vi "Generate Report work with Zee.vi"(6 "Graph Properties":T2(array[cluster])=[{"Plot Traces"=[{"Color Box"=4652800, "Boolean"=TRUE, "List 2"=5, "Boolean 2"=FALSE, "Boolean 3"=FALSE, "Offset"=0.0, "Gain"=1.0}, {"Color Box"=4467455, "Boolean"=TRUE, "List 2"=13, "Boolean 2"=TRUE, "Boolean 3"=FALSE, "Offset"=0.0, "Gain"=1.0}, {"Color Box"=16722474, "Boolean"=TRUE, "List 2"=21, "Boolean 2"=TRUE, "Boolean 3"=FALSE, "Offset"=0.0, "Gain"=1.0}], "Gain Calculations"={"Threshold Trace"=5, "Min Thresh/%"=0.2, "Max Thresh/%"=0.8, "Gain calculated by dividing"=13, "Gain Range"=enum."Best Est", "Pre-peak-ms"=30.0, "by"=5}, "Impulse Plane"=enum."Yaw", "Impulse Direction"=TRUE}, {"Plot Traces"=[{"Color Box"=4652800, "Boolean"=TRUE, "List 2"=5, "Boolean 2"=TRUE, "Boolean 3"=FALSE, "Offset"=0.0, "Gain"=1.0}, {"Color Box"=1966335, "Boolean"=TRUE, "List 2"=13, "Boolean 2"=FALSE, "Boolean 3"=FALSE, "Offset"=0.0, "Gain"=1.0}, {"Color Box"=16722474, "Boolean"=TRUE, "List 2"=21, "Boolean 2"=FALSE, "Boolean 3"=FALSE, "Offset"=0.0, "Gain"=1.0}], "Gain Calculations"={"Threshold Trace"=5, "Min Thresh/%"=0.2, "Max Thresh/%"=0.8, "Gain calculated by dividing"=13, "Gain Range"=enum."Best Est", "Pre-peak-ms"=30.0, "by"=5}, "Impulse Plane"=enum."Yaw", "Impulse Direction"=FALSE}, {"Plot Traces"=[{"Color Box"=4652800, "Boolean"=TRUE, "List 2"=5, "Boolean 2"=FALSE, "Boolean 3"=FALSE, "Offset"=0.0, "Gain"=1.0}, {"Color Box"=1966335, "Boolean"=TRUE, "List 2"=13, "Boolean 2"=TRUE, "Boolean 3"=FALSE, "Offset"=0.0, "Gain"=1.0}, {"Color Box"=16722474, "Boolean"=TRUE, "List 2"=21, "Boolean 2"=TRUE, "Boolean 3"=FALSE, "Offset"=0.0, "Gain"=1.0}], "Gain Calculations"={"Threshold Trace"=5, "Min Thresh/%"=0.2, "Max Thresh/%"=0.8, "Gain calculated by dividing"=21, "Gain Range"=enum."Best Est", "Pre-peak-ms"=30.0, "by"=5}, "Impulse Plane"=enum."Yaw", "Impulse Direction"=TRUE}, {"Plot Traces"=[{"Color Box"=4652800, "Boolean"=TRUE, "List 2"=5, "Boolean 2"=TRUE, "Boolean 3"=FALSE, "Offset"=0.0, "Gain"=1.0}, {"Color Box"=1966335, "Boolean"=TRUE, "List 2"=13, "Boolean 2"=FALSE, "Boolean 3"=FALSE, "Offset"=0.0, "Gain"=1.0}, {"Color Box"=16722474, "Boolean"=TRUE, "List 2"=21, "Boolean 2"=FALSE, "Boolean 3"=FALSE, "Offset"=0.0, "Gain"=1.0}], "Gain Calculations"={"Threshold Trace"=5, "Min Thresh/%"=0.2, "Max Thresh/%"=0.8, "Gain calculated by dividing"=21, "Gain Range"=enum."Best Est", "Pre-peak-ms"=30.0, "by"=5}, "Impulse Plane"=enum."Yaw", "Impulse Direction"=FALSE}, {"Plot Traces"=[{"Color Box"=4652800, "Boolean"=TRUE, "List 2"=4, "Boolean 2"=FALSE, "Boolean 3"=FALSE, "Offset"=0.0, "Gain"=1.0}, {"Color Box"=1966335, "Boolean"=TRUE, "List 2"=12, "Boolean 2"=TRUE, "Boolean 3"=FALSE, "Offset"=0.0, "Gain"=1.0}, {"Color Box"=16722474, "Boolean"=TRUE, "List 2"=20, "Boolean 2"=TRUE, "Boolean 3"=FALSE, "Offset"=0.0, "Gain"=1.0}], "Gain Calculations"={"Threshold Trace"=4, "Min Thresh/%"=0.2, "Max Thresh/%"=0.8, "Gain calculated by dividing"=12, "Gain Range"=enum."Best Est", "Pre-peak-ms"=30.0, "by"=4}, "Impulse Plane"=enum."Pitch", "Impulse Direction"=TRUE}, {"Plot Traces"=[{"Color Box"=4652800, "Boolean"=TRUE, "List 2"=4, "Boolean 2"=TRUE, "Boolean 3"=FALSE, "Offset"=0.0, "Gain"=1.0}, {"Color Box"=1966335, "Boolean"=TRUE, "List 2"=12, "Boolean 2"=FALSE, "Boolean 3"=FALSE, "Offset"=0.0, "Gain"=1.0}, {"Color Box"=16722474, "Boolean"=TRUE, "List 2"=20, "Boolean 2"=FALSE, "Boolean 3"=FALSE, "Offset"=0.0, "Gain"=1.0}], "Gain Calculations"={"Threshold Trace"=4, "Min Thresh/%"=0.2, "Max Thresh/%"=0.8, "Gain calculated by dividing"=12, "Gain Range"=enum."Best Est", "Pre-peak-ms"=30.0, "by"=4}, "Impulse Plane"=enum."Pitch", "Impulse Direction"=FALSE}, {"Plot Traces"=[{"Color Box"=4652800, "Boolean"=TRUE, "List 2"=4, "Boolean 2"=FALSE, "Boolean 3"=FALSE, "Offset"=0.0, "Gain"=1.0}, {"Color Box"=16860, "Boolean"=TRUE, "List 2"=12, "Boolean 2"=TRUE, "Boolean 3"=FALSE, "Offset"=0.0, "Gain"=1.0}, {"Color Box"=16716346, "Boolean"=TRUE, "List 2"=20, "Boolean 2"=TRUE, "Boolean 3"=FALSE, "Offset"=0.0, "Gain"=1.0}], "Gain Calculations"={"Threshold Trace"=4, "Min Thresh/%"=0.2, "Max Thresh/%"=0.8, "Gain calculated by dividing"=20, "Gain Range"=enum."Best Est", "Pre-peak-ms"=30.0, "by"=4}, "Impulse Plane"=enum."Pitch", "Impulse Direction"=TRUE}, {"Plot Traces"=[{"Color Box"=4652800, "Boolean"=TRUE, "List 2"=4, "Boolean 2"=TRUE, "Boolean 3"=FALSE, "Offset"=0.0, "Gain"=1.0}, {"Color Box"=4349695, "Boolean"=TRUE, "List 2"=12, "Boolean 2"=FALSE, "Boolean 3"=FALSE, "Offset"=0.0, "Gain"=1.0}, {"Color Box"=16716346, "Boolean"=TRUE, "List 2"=20, "Boolean 2"=FALSE, "Boolean 3"=FALSE, "Offset"=0.0, "Gain"=1.0}], "Gain Calculations"={"Threshold Trace"=4, "Min Thresh/%"=0.2, "Max Thresh/%"=0.8, "Gain calculated by dividing"=20, "Gain Range"=enum."Best Est", "Pre-peak-ms"=30.0, "by"=4}, "Impulse Plane"=enum."Pitch", "Impulse Direction"=FALSE}, {"Plot Traces"=[{"Color Box"=4652800, "Boolean"=TRUE, "List 2"=3, "Boolean 2"=FALSE, "Boolean 3"=FALSE, "Offset"=0.0, "Gain"=1.0}, {"Color Box"=4349695, "Boolean"=TRUE, "List 2"=11, "Boolean 2"=TRUE, "Boolean 3"=FALSE, "Offset"=0.0, "Gain"=1.0}, {"Color Box"=16716346, "Boolean"=TRUE, "List 2"=19, "Boolean 2"=TRUE, "Boolean 3"=FALSE, "Offset"=0.0, "Gain"=1.0}], "Gain Calculations"={"Threshold Trace"=3, "Min Thresh/%"=0.2, "Max Thresh/%"=0.8, "Gain calculated by dividing"=11, "Gain Range"=enum."Best Est", "Pre-peak-ms"=30.0, "by"=3}, "Impulse Plane"=enum."Roll", "Impulse Direction"=TRUE}, {"Plot Traces"=[{"Color Box"=4652800, "Boolean"=TRUE, "List 2"=3, "Boolean 2"=TRUE, "Boolean 3"=FALSE, "Offset"=0.0, "Gain"=1.0}, {"Color Box"=4349695, "Boolean"=TRUE, "List 2"=11, "Boolean 2"=FALSE, "Boolean 3"=FALSE, "Offset"=0.0, "Gain"=1.0}, {"Color Box"=16716346, "Boolean"=TRUE, "List 2"=19, "Boolean 2"=FALSE, "Boolean 3"=FALSE, "Offset"=0.0, "Gain"=1.0}], "Gain Calculations"={"Threshold Trace"=3, "Min Thresh/%"=0.2, "Max Thresh/%"=0.8, "Gain calculated by dividing"=11, "Gain Range"=enum."Best Est", "Pre-peak-ms"=30.0, "by"=3}, "Impulse Plane"=enum."Roll", "Impulse Direction"=FALSE}, {"Plot Traces"=[{"Color Box"=4652800, "Boolean"=TRUE, "List 2"=3, "Boolean 2"=FALSE, "Boolean 3"=FALSE, "Offset"=0.0, "Gain"=1.0}, {"Color Box"=4349695, "Boolean"=TRUE, "List 2"=11, "Boolean 2"=TRUE, "Boolean 3"=FALSE, "Offset"=0.0, "Gain"=1.0}, {"Color Box"=16716346, "Boolean"=TRUE, "List 2"=19, "Boolean 2"=TRUE, "Boolean 3"=FALSE, "Offset"=0.0, "Gain"=1.0}], "Gain Calculations"={"Threshold Trace"=3, "Min Thresh/%"=0.2, "Max Thresh/%"=0.8, "Gain calculated by dividing"=19, "Gain Range"=enum."Best Est", "Pre-peak-ms"=30.0, "by"=3}, "Impulse Plane"=enum."Roll", "Impulse Direction"=TRUE}, {"Plot Traces"=[{"Color Box"=4652800, "Boolean"=TRUE, "List 2"=3, "Boolean 2"=TRUE, "Boolean 3"=FALSE, "Offset"=0.0, "Gain"=1.0}, {"Color Box"=4349695, "Boolean"=TRUE, "List 2"=11, "Boolean 2"=FALSE, "Boolean 3"=FALSE, "Offset"=0.0, "Gain"=1.0}, {"Color Box"=16716346, "Boolean"=TRUE, "List 2"=19, "Boolean 2"=FALSE, "Boolean 3"=FALSE, "Offset"=0.0, "Gain"=1.0}], "Gain Calculations"={"Threshold Trace"=3, "Min Thresh/%"=0.2, "Max Thresh/%"=0.8, "Gain calculated by dividing"=19, "Gain Range"=enum."Best Est", "Pre-peak-ms"=30.0, "by"=3}, "Impulse Plane"=enum."Roll", "Impulse Direction"=FALSE}, {"Plot Traces"=[{"Color Box"=4652800, "Boolean"=TRUE, "List 2"=4, "Boolean 2"=TRUE, "Boolean 3"=FALSE, "Offset"=0.0, "Gain"=1.0}, {"Color Box"=4349695, "Boolean"=TRUE, "List 2"=12, "Boolean 2"=FALSE, "Boolean 3"=FALSE, "Offset"=0.0, "Gain"=1.0}, {"Color Box"=16716346, "Boolean"=TRUE, "List 2"=20, "Boolean 2"=FALSE, "Boolean 3"=FALSE, "Offset"=0.0, "Gain"=1.0}], "Gain Calculations"={"Threshold Trace"=4, "Min Thresh/%"=0.2, "Max Thresh/%"=0.8, "Gain calculated by dividing"=12, "Gain Range"=enum."Best Est", "Pre-peak-ms"=30.0, "by"=4}, "Impulse Plane"=enum."LARP", "Impulse Direction"=TRUE}, {"Plot Traces"=[{"Color Box"=4652800, "Boolean"=TRUE, "List 2"=4, "Boolean 2"=FALSE, "Boolean 3"=FALSE, "Offset"=0.0, "Gain"=1.0}, {"Color Box"=4349695, "Boolean"=TRUE, "List 2"=12, "Boolean 2"=TRUE, "Boolean 3"=FALSE, "Offset"=0.0, "Gain"=1.0}, {"Color Box"=16716346, "Boolean"=TRUE, "List 2"=20, "Boolean 2"=TRUE, "Boolean 3"=FALSE, "Offset"=0.0, "Gain"=1.0}], "Gain Calculations"={"Threshold Trace"=4, "Min Thresh/%"=0.2, "Max Thresh/%"=0.8, "Gain calculated by dividing"=12, "Gain Range"=enum."Best Est", "Pre-peak-ms"=30.0, "by"=4}, "Impulse Plane"=enum."LARP", "Impulse Direction"=FALSE}, {"Plot Traces"=[{"Color Box"=4652800, "Boolean"=TRUE, "List 2"=4, "Boolean 2"=TRUE, "Boolean 3"=FALSE, "Offset"=0.0, "Gain"=1.0}, {"Color Box"=4349695, "Boolean"=TRUE, "List 2"=12, "Boolean 2"=FALSE, "Boolean 3"=FALSE, "Offset"=0.0, "Gain"=1.0}, {"Color Box"=16716346, "Boolean"=TRUE, "List 2"=20, "Boolean 2"=FALSE, "Boolean 3"=FALSE, "Offset"=0.0, "Gain"=1.0}], "Gain Calculations"={"Threshold Trace"=4, "Min Thresh/%"=0.2, "Max Thresh/%"=0.8, "Gain calculated by dividing"=20, "Gain Range"=enum."Best Est", "Pre-peak-ms"=30.0, "by"=4}, "Impulse Plane"=enum."LARP", "Impulse Direction"=TRUE}, {"Plot Traces"=[{"Color Box"=4652800, "Boolean"=TRUE, "List 2"=4, "Boolean 2"=FALSE, "Boolean 3"=FALSE, "Offset"=0.0, "Gain"=1.0}, {"Color Box"=4349695, "Boolean"=TRUE, "List 2"=12, "Boolean 2"=TRUE, "Boolean 3"=FALSE, "Offset"=0.0, "Gain"=1.0}, {"Color Box"=16716346, "Boolean"=TRUE, "List 2"=20, "Boolean 2"=TRUE, "Boolean 3"=FALSE, "Offset"=0.0, "Gain"=1.0}], "Gain Calculations"={"Threshold Trace"=4, "Min Thresh/%"=0.2, "Max Thresh/%"=0.8, "Gain calculated by dividing"=20, "Gain Range"=enum."Best Est", "Pre-peak-ms"=30.0, "by"=4}, "Impulse Plane"=enum."LARP", "Impulse Direction"=FALSE}, {"Plot Traces"=[{"Color Box"=4652800, "Boolean"=TRUE, "List 2"=3, "Boolean 2"=FALSE, "Boolean 3"=FALSE, "Offset"=0.0, "Gain"=1.0}, {"Color Box"=4349695, "Boolean"=TRUE, "List 2"=11, "Boolean 2"=TRUE, "Boolean 3"=FALSE, "Offset"=0.0, "Gain"=1.0}, {"Color Box"=16716346, "Boolean"=TRUE, "List 2"=19, "Boolean 2"=TRUE, "Boolean 3"=FALSE, "Offset"=0.0, "Gain"=1.0}], "Gain Calculations"={"Threshold Trace"=3, "Min Thresh/%"=0.2, "Max Thresh/%"=0.8, "Gain calculated by dividing"=11, "Gain Range"=enum."Best Est", "Pre-peak-ms"=30.0, "by"=3}, "Impulse Plane"=enum."LARP", "Impulse Direction"=TRUE}, {"Plot Traces"=[{"Color Box"=4652800, "Boolean"=TRUE, "List 2"=3, "Boolean 2"=TRUE, "Boolean 3"=FALSE, "Offset"=0.0, "Gain"=1.0}, {"Color Box"=4349695, "Boolean"=TRUE, "List 2"=11, "Boolean 2"=FALSE, "Boolean 3"=FALSE, "Offset"=0.0, "Gain"=1.0}, {"Color Box"=16716346, "Boolean"=TRUE, "List 2"=19, "Boolean 2"=FALSE, "Boolean 3"=FALSE, "Offset"=0.0, "Gain"=1.0}], "Gain Calculations"={"Threshold Trace"=3, "Min Thresh/%"=0.2, "Max Thresh/%"=0.8, "Gain calculated by dividing"=11, "Gain Range"=enum."Best Est", "Pre-peak-ms"=30.0, "by"=3}, "Impulse Plane"=enum."LARP", "Impulse Direction"=FALSE}, {"Plot Traces"=[{"Color Box"=4652800, "Boolean"=TRUE, "List 2"=3, "Boolean 2"=FALSE, "Boolean 3"=FALSE, "Offset"=0.0, "Gain"=1.0}, {"Color Box"=4349695, "Boolean"=TRUE, "List 2"=11, "Boolean 2"=TRUE, "Boolean 3"=FALSE, "Offset"=0.0, "Gain"=1.0}, {"Color Box"=16716346, "Boolean"=TRUE, "List 2"=19, "Boolean 2"=TRUE, "Boolean 3"=FALSE, "Offset"=0.0, "Gain"=1.0}], "Gain Calculations"={"Threshold Trace"=3, "Min Thresh/%"=0.2, "Max Thresh/%"=0.8, "Gain calculated by dividing"=19, "Gain Range"=enum."Best Est", "Pre-peak-ms"=30.0, "by"=3}, "Impulse Plane"=enum."LARP", "Impulse Direction"=TRUE}, {"Plot Traces"=[{"Color Box"=4652800, "Boolean"=TRUE, "List 2"=3, "Boolean 2"=TRUE, "Boolean 3"=FALSE, "Offset"=0.0, "Gain"=1.0}, {"Color Box"=4349695, "Boolean"=TRUE, "List 2"=11, "Boolean 2"=FALSE, "Boolean 3"=FALSE, "Offset"=0.0, "Gain"=1.0}, {"Color Box"=16716346, "Boolean"=TRUE, "List 2"=19, "Boolean 2"=FALSE, "Boolean 3"=FALSE, "Offset"=0.0, "Gain"=1.0}], "Gain Calculations"={"Threshold Trace"=3, "Min Thresh/%"=0.2, "Max Thresh/%"=0.8, "Gain calculated by dividing"=19, "Gain Range"=enum."Best Est", "Pre-peak-ms"=30.0, "by"=3}, "Impulse Plane"=enum."LARP", "Impulse Direction"=FALSE}, {"Plot Traces"=[{"Color Box"=4652800, "Boolean"=TRUE, "List 2"=4, "Boolean 2"=FALSE, "Boolean 3"=FALSE, "Offset"=0.0, "Gain"=1.0}, {"Color Box"=4349695, "Boolean"=TRUE, "List 2"=12, "Boolean 2"=TRUE, "Boolean 3"=FALSE, "Offset"=0.0, "Gain"=1.0}, {"Color Box"=16716346, "Boolean"=TRUE, "List 2"=20, "Boolean 2"=TRUE, "Boolean 3"=FALSE, "Offset"=0.0, "Gain"=1.0}], "Gain Calculations"={"Threshold Trace"=4, "Min Thresh/%"=0.2, "Max Thresh/%"=0.8, "Gain calculated by dividing"=12, "Gain Range"=enum."Best Est", "Pre-peak-ms"=30.0, "by"=4}, "Impulse Plane"=enum."RALP", "Impulse Direction"=TRUE}, {"Plot Traces"=[{"Color Box"=4652800, "Boolean"=TRUE, "List 2"=4, "Boolean 2"=TRUE, "Boolean 3"=FALSE, "Offset"=0.0, "Gain"=1.0}, {"Color Box"=4349695, "Boolean"=TRUE, "List 2"=12, "Boolean 2"=FALSE, "Boolean 3"=FALSE, "Offset"=0.0, "Gain"=1.0}, {"Color Box"=16716346, "Boolean"=TRUE, "List 2"=20, "Boolean 2"=FALSE, "Boolean 3"=FALSE, "Offset"=0.0, "Gain"=1.0}], "Gain Calculations"={"Threshold Trace"=4, "Min Thresh/%"=0.2, "Max Thresh/%"=0.8, "Gain calculated by dividing"=12, "Gain Range"=enum."Best Est", "Pre-peak-ms"=30.0, "by"=4}, "Impulse Plane"=enum."RALP", "Impulse Direction"=FALSE}, {"Plot Traces"=[{"Color Box"=4652800, "Boolean"=TRUE, "List 2"=4, "Boolean 2"=FALSE, "Boolean 3"=FALSE, "Offset"=0.0, "Gain"=1.0}, {"Color Box"=4349695, "Boolean"=TRUE, "List 2"=12, "Boolean 2"=TRUE, "Boolean 3"=FALSE, "Offset"=0.0, "Gain"=1.0}, {"Color Box"=16716346, "Boolean"=TRUE, "List 2"=20, "Boolean 2"=TRUE, "Boolean 3"=FALSE, "Offset"=0.0, "Gain"=1.0}], "Gain Calculations"={"Threshold Trace"=4, "Min Thresh/%"=0.2, "Max Thresh/%"=0.8, "Gain calculated by dividing"=20, "Gain Range"=enum."Best Est", "Pre-peak-ms"=30.0, "by"=4}, "Impulse Plane"=enum."RALP", "Impulse Direction"=TRUE}, {"Plot Traces"=[{"Color Box"=4652800, "Boolean"=TRUE, "List 2"=4, "Boolean 2"=TRUE, "Boolean 3"=FALSE, "Offset"=0.0, "Gain"=1.0}, {"Color Box"=4349695, "Boolean"=TRUE, "List 2"=12, "Boolean 2"=FALSE, "Boolean 3"=FALSE, "Offset"=0.0, "Gain"=1.0}, {"Color Box"=16716346, "Boolean"=TRUE, "List 2"=20, "Boolean 2"=FALSE, "Boolean 3"=FALSE, "Offset"=0.0, "Gain"=1.0}], "Gain Calculations"={"Threshold Trace"=4, "Min Thresh/%"=0.2, "Max Thresh/%"=0.8, "Gain calculated by dividing"=20, "Gain Range"=enum."Best Est", "Pre-peak-ms"=30.0, "by"=4}, "Impulse Plane"=enum."RALP", "Impulse Direction"=FALSE}, {"Plot Traces"=[{"Color Box"=4652800, "Boolean"=TRUE, "List 2"=3, "Boolean 2"=FALSE, "Boolean 3"=FALSE, "Offset"=0.0, "Gain"=1.0}, {"Color Box"=4349695, "Boolean"=TRUE, "List 2"=11, "Boolean 2"=TRUE, "Boolean 3"=FALSE, "Offset"=0.0, "Gain"=1.0}, {"Color Box"=16716346, "Boolean"=TRUE, "List 2"=19, "Boolean 2"=TRUE, "Boolean 3"=FALSE, "Offset"=0.0, "Gain"=1.0}], "Gain Calculations"={"Threshold Trace"=3, "Min Thresh/%"=0.2, "Max Thresh/%"=0.8, "Gain calculated by dividing"=11, "Gain Range"=enum."Best Est", "Pre-peak-ms"=30.0, "by"=3}, "Impulse Plane"=enum."RALP", "Impulse Direction"=TRUE}, {"Plot Traces"=[{"Color Box"=4652800, "Boolean"=TRUE, "List 2"=3, "Boolean 2"=TRUE, "Boolean 3"=FALSE, "Offset"=0.0, "Gain"=1.0}, {"Color Box"=4349695, "Boolean"=TRUE, "List 2"=11, "Boolean 2"=FALSE, "Boolean 3"=FALSE, "Offset"=0.0, "Gain"=1.0}, {"Color Box"=16716346, "Boolean"=TRUE, "List 2"=19, "Boolean 2"=FALSE, "Boolean 3"=FALSE, "Offset"=0.0, "Gain"=1.0}], "Gain Calculations"={"Threshold Trace"=3, "Min Thresh/%"=0.2, "Max Thresh/%"=0.8, "Gain calculated by dividing"=11, "Gain Range"=enum."Best Est", "Pre-peak-ms"=30.0, "by"=3}, "Impulse Plane"=enum."RALP", "Impulse Direction"=FALSE}, {"Plot Traces"=[{"Color Box"=4652800, "Boolean"=TRUE, "List 2"=3, "Boolean 2"=FALSE, "Boolean 3"=FALSE, "Offset"=0.0, "Gain"=1.0}, {"Color Box"=4349695, "Boolean"=TRUE, "List 2"=11, "Boolean 2"=TRUE, "Boolean 3"=FALSE, "Offset"=0.0, "Gain"=1.0}, {"Color Box"=16716346, "Boolean"=TRUE, "List 2"=19, "Boolean 2"=TRUE, "Boolean 3"=FALSE, "Offset"=0.0, "Gain"=1.0}], "Gain Calculations"={"Threshold Trace"=3, "Min Thresh/%"=0.2, "Max Thresh/%"=0.8, "Gain calculated by dividing"=19, "Gain Range"=enum."Best Est", "Pre-peak-ms"=30.0, "by"=3}, "Impulse Plane"=enum."RALP", "Impulse Direction"=TRUE}, {"Plot Traces"=[{"Color Box"=4652800, "Boolean"=TRUE, "List 2"=3, "Boolean 2"=TRUE, "Boolean 3"=FALSE, "Offset"=0.0, "Gain"=1.0}, {"Color Box"=4349695, "Boolean"=TRUE, "List 2"=11, "Boolean 2"=FALSE, "Boolean 3"=FALSE, "Offset"=0.0, "Gain"=1.0}, {"Color Box"=16716346, "Boolean"=TRUE, "List 2"=19, "Boolean 2"=FALSE, "Boolean 3"=FALSE, "Offset"=0.0, "Gain"=1.0}], "Gain Calculations"={"Threshold Trace"=3, "Min Thresh/%"=0.2, "Max Thresh/%"=0.8, "Gain calculated by dividing"=19, "Gain Range"=enum."Best Est", "Pre-peak-ms"=30.0, "by"=3}, "Impulse Plane"=enum."RALP", "Impulse Direction"=FALSE}, {"Plot Traces"=[{"Color Box"=4652800, "Boolean"=TRUE, "List 2"=6, "Boolean 2"=FALSE, "Boolean 3"=FALSE, "Offset"=0.0, "Gain"=1.0}, {"Color Box"=16733696, "Boolean"=TRUE, "List 2"=14, "Boolean 2"=TRUE, "Boolean 3"=FALSE, "Offset"=0.0, "Gain"=1.0}, {"Color Box"=393436, "Boolean"=TRUE, "List 2"=22, "Boolean 2"=TRUE, "Boolean 3"=FALSE, "Offset"=0.0, "Gain"=1.0}], "Gain Calculations"={"Threshold Trace"=6, "Min Thresh/%"=0.2, "Max Thresh/%"=0.8, "Gain calculated by dividing"=14, "Gain Range"=enum."Best Est", "Pre-peak-ms"=30.0, "by"=6}, "Impulse Plane"=enum."LARP", "Impulse Direction"=TRUE}, {"Plot Traces"=[{"Color Box"=4652800, "Boolean"=TRUE, "List 2"=6, "Boolean 2"=TRUE, "Boolean 3"=FALSE, "Offset"=0.0, "Gain"=1.0}, {"Color Box"=16733696, "Boolean"=TRUE, "List 2"=14, "Boolean 2"=FALSE, "Boolean 3"=FALSE, "Offset"=0.0, "Gain"=1.0}, {"Color Box"=393436, "Boolean"=TRUE, "List 2"=22, "Boolean 2"=FALSE, "Boolean 3"=FALSE, "Offset"=0.0, "Gain"=1.0}], "Gain Calculations"={"Threshold Trace"=6, "Min Thresh/%"=0.2, "Max Thresh/%"=0.8, "Gain calculated by dividing"=14, "Gain Range"=enum."Best Est", "Pre-peak-ms"=30.0, "by"=6}, "Impulse Plane"=enum."LARP", "Impulse Direction"=FALSE}, {"Plot Traces"=[{"Color Box"=4652800, "Boolean"=TRUE, "List 2"=6, "Boolean 2"=FALSE, "Boolean 3"=FALSE, "Offset"=0.0, "Gain"=1.0}, {"Color Box"=16733696, "Boolean"=TRUE, "List 2"=14, "Boolean 2"=TRUE, "Boolean 3"=FALSE, "Offset"=0.0, "Gain"=1.0}, {"Color Box"=393436, "Boolean"=TRUE, "List 2"=22, "Boolean 2"=TRUE, "Boolean 3"=FALSE, "Offset"=0.0, "Gain"=1.0}], "Gain Calculations"={"Threshold Trace"=6, "Min Thresh/%"=0.2, "Max Thresh/%"=0.8, "Gain calculated by dividing"=22, "Gain Range"=enum."Best Est", "Pre-peak-ms"=30.0, "by"=6}, "Impulse Plane"=enum."LARP", "Impulse Direction"=TRUE}, {"Plot Traces"=[{"Color Box"=4652800, "Boolean"=TRUE, "List 2"=6, "Boolean 2"=TRUE, "Boolean 3"=FALSE, "Offset"=0.0, "Gain"=1.0}, {"Color Box"=16733696, "Boolean"=TRUE, "List 2"=14, "Boolean 2"=FALSE, "Boolean 3"=FALSE, "Offset"=0.0, "Gain"=1.0}, {"Color Box"=393436, "Boolean"=TRUE, "List 2"=22, "Boolean 2"=FALSE, "Boolean 3"=FALSE, "Offset"=0.0, "Gain"=1.0}], "Gain Calculations"={"Threshold Trace"=6, "Min Thresh/%"=0.2, "Max Thresh/%"=0.8, "Gain calculated by dividing"=22, "Gain Range"=enum."Best Est", "Pre-peak-ms"=30.0, "by"=6}, "Impulse Plane"=enum."LARP", "Impulse Direction"=FALSE}, {"Plot Traces"=[{"Color Box"=4652800, "Boolean"=TRUE, "List 2"=7, "Boolean 2"=FALSE, "Boolean 3"=FALSE, "Offset"=0.0, "Gain"=1.0}, {"Color Box"=16733696, "Boolean"=TRUE, "List 2"=15, "Boolean 2"=TRUE, "Boolean 3"=FALSE, "Offset"=0.0, "Gain"=1.0}, {"Color Box"=393436, "Boolean"=TRUE, "List 2"=23, "Boolean 2"=TRUE, "Boolean 3"=FALSE, "Offset"=0.0, "Gain"=1.0}], "Gain Calculations"={"Threshold Trace"=7, "Min Thresh/%"=0.2, "Max Thresh/%"=0.8, "Gain calculated by dividing"=15, "Gain Range"=enum."Best Est", "Pre-peak-ms"=30.0, "by"=7}, "Impulse Plane"=enum."RALP", "Impulse Direction"=TRUE}, {"Plot Traces"=[{"Color Box"=4652800, "Boolean"=TRUE, "List 2"=7, "Boolean 2"=TRUE, "Boolean 3"=FALSE, "Offset"=0.0, "Gain"=1.0}, {"Color Box"=16733696, "Boolean"=TRUE, "List 2"=15, "Boolean 2"=FALSE, "Boolean 3"=FALSE, "Offset"=0.0, "Gain"=1.0}, {"Color Box"=393436, "Boolean"=TRUE, "List 2"=23, "Boolean 2"=FALSE, "Boolean 3"=FALSE, "Offset"=0.0, "Gain"=1.0}], "Gain Calculations"={"Threshold Trace"=7, "Min Thresh/%"=0.2, "Max Thresh/%"=0.8, "Gain calculated by dividing"=15, "Gain Range"=enum."Best Est", "Pre-peak-ms"=30.0, "by"=7}, "Impulse Plane"=enum."RALP", "Impulse Direction"=FALSE}, {"Plot Traces"=[{"Color Box"=4652800, "Boolean"=TRUE, "List 2"=7, "Boolean 2"=FALSE, "Boolean 3"=FALSE, "Offset"=0.0, "Gain"=1.0}, {"Color Box"=16733696, "Boolean"=TRUE, "List 2"=15, "Boolean 2"=TRUE, "Boolean 3"=FALSE, "Offset"=0.0, "Gain"=1.0}, {"Color Box"=393436, "Boolean"=TRUE, "List 2"=23, "Boolean 2"=TRUE, "Boolean 3"=FALSE, "Offset"=0.0, "Gain"=1.0}], "Gain Calculations"={"Threshold Trace"=7, "Min Thresh/%"=0.2, "Max Thresh/%"=0.8, "Gain calculated by dividing"=23, "Gain Range"=enum."Best Est", "Pre-peak-ms"=30.0, "by"=7}, "Impulse Plane"=enum."RALP", "Impulse Direction"=TRUE}, {"Plot Traces"=[{"Color Box"=4652800, "Boolean"=TRUE, "List 2"=7, "Boolean 2"=TRUE, "Boolean 3"=FALSE, "Offset"=0.0, "Gain"=1.0}, {"Color Box"=16733696, "Boolean"=TRUE, "List 2"=15, "Boolean 2"=FALSE, "Boolean 3"=FALSE, "Offset"=0.0, "Gain"=1.0}, {"Color Box"=393436, "Boolean"=TRUE, "List 2"=23, "Boolean 2"=FALSE, "Boolean 3"=FALSE, "Offset"=0.0, "Gain"=1.0}], "Gain Calculations"={"Threshold Trace"=7, "Min Thresh/%"=0.2, "Max Thresh/%"=0.8, "Gain calculated by dividing"=23, "Gain Range"=enum."Best Est", "Pre-peak-ms"=30.0, "by"=7}, "Impulse Plane"=enum."RALP", "Impulse Direction"=FALSE}] {"Gain Calculations"."by" items=["Hx Position-in-Head", "Hy Position-in-Head", "Hz Position-in-Head", "Hx Velocity-in-Head", "Hy Velocity-in-Head", "Hz Velocity-in-Head", "Hl Velocity-in-Head", "Hr Velocity-in-Head", "Lx Position-in-Head", "Ly Position-in-Head", "Lz Position-in-Head", "Lx Velocity-in-Head", "Ly Velocity-in-Head", "Lz Velocity-in-Head", "Ll Velocity-in-Head", "Lr Velocity-in-Head", "Rx Position-in-Head", "Ry Position-in-Head", "Rz Position-in-Head", "Rx Velocity-in-Head", "Ry Velocity-in-Head", "Rz Velocity-in-Head", "Rl Velocity-in-Head", "Rr Velocity-in-Head", "Button", "Ascension X", "Ascension X Vel", "Ascension Y", "Ascension Y Vel", "Ascension Z", "Ascension Z Vel", " ", "Lx Velocity-in-Eye", "Ly Velocity-in-Eye", "Lz Velocity-in-Eye"]; "Gain Calculations"."Pre-peak-ms" format="%.2f"; "Gain Calculations"."Gain calculated by dividing" items=["Hx Position-in-Head", "Hy Position-in-Head", "Hz Position-in-Head", "Hx Velocity-in-Head", "Hy Velocity-in-Head", "Hz Velocity-in-Head", "Hl Velocity-in-Head", "Hr Velocity-in-Head", "Lx Position-in-Head", "Ly Position-in-Head", "Lz Position-in-Head", "Lx Velocity-in-Head", "Ly Velocity-in-Head", "Lz Velocity-in-Head", "Ll Velocity-in-Head", "Lr Velocity-in-Head", "Rx Position-in-Head", "Ry Position-in-Head", "Rz Position-in-Head", "Rx Velocity-in-Head", "Ry Velocity-in-Head", "Rz Velocity-in-Head", "Rl Velocity-in-Head", "Rr Velocity-in-Head", "Button", "Ascension X", "Ascension X Vel", "Ascension Y", "Ascension Y Vel", "Ascension Z", "Ascension Z Vel", " ", "Lx Velocity-in-Eye", "Ly Velocity-in-Eye", "Lz Velocity-in-Eye"]; "Gain Calculations"."Max Thresh/%" format="%.2f"; "Gain Calculations"."Min Thresh/%" format="%.2f"; "Gain Calculations"."Threshold Trace" items=["Hx Position-in-Head", "Hy Position-in-Head", "Hz Position-in-Head", "Hx Velocity-in-Head", "Hy Velocity-in-Head", "Hz Velocity-in-Head", "Hl Velocity-in-Head", "Hr Velocity-in-Head", "Lx Position-in-Head", "Ly Position-in-Head", "Lz Position-in-Head", "Lx Velocity-in-Head", "Ly Velocity-in-Head", "Lz Velocity-in-Head", "Ll Velocity-in-Head", "Lr Velocity-in-Head", "Rx Position-in-Head", "Ry Position-in-Head", "Rz Position-in-Head", "Rx Velocity-in-Head", "Ry Velocity-in-Head", "Rz Velocity-in-Head", "Rl Velocity-in-Head", "Rr Velocity-in-Head", "Button", "Ascension X", "Ascension X Vel", "Ascension Y", "Ascension Y Vel", "Ascension Z", "Ascension Z Vel", " ", "Lx Velocity-in-Eye", "Ly Velocity-in-Eye", "Lz Velocity-in-Eye"]; "Plot Traces"."Gain" format="%.1f"; "Plot Traces"."Offset" format="%.1f"; "Plot Traces"."List 2" items=["Hx Position-in-Head", "Hy Position-in-Head", "Hz Position-in-Head", "Hx Velocity-in-Head", "Hy Velocity-in-Head", "Hz Velocity-in-Head", "Hl Velocity-in-Head", "Hr Velocity-in-Head", "Lx Position-in-Head", "Ly Position-in-Head", "Lz Position-in-Head", "Lx Velocity-in-Head", "Ly Velocity-in-Head", "Lz Velocity-in-Head", "Ll Velocity-in-Head", "Lr Velocity-in-Head", "Rx Position-in-Head", "Ry Position-in-Head", "Rz Position-in-Head", "Rx Velocity-in-Head", "Ry Velocity-in-Head", "Rz Velocity-in-Head", "Rl Velocity-in-Head", "Rr Velocity-in-Head", "Button", "Ascension X", "Ascension X Vel", "Ascension Y", "Ascension Y Vel", "Ascension Z", "Ascension Z Vel", " ", "Lx Velocity-in-Eye", "Ly Velocity-in-Eye", "Lz Velocity-in-Eye"]}, 8 "Impulse Positions":T4(array[cluster])=[{"Start"=4649, "End"=4716, "Impulse Plane"=enum."Yaw", "Impulse Direction +ve?"=FALSE, "Time offset"=0, "Amplitude offset"=0.0}, {"Start"=7434, "End"=7492, "Impulse Plane"=enum."Yaw", "Impulse Direction +ve?"=TRUE, "Time offset"=0, "Amplitude offset"=0.0}, {"Start"=8253, "End"=8319, "Impulse Plane"=enum."Yaw", "Impulse Direction +ve?"=FALSE, "Time offset"=0, "Amplitude offset"=0.0}, {"Start"=9839, "End"=9899, "Impulse Plane"=enum."Yaw", "Impulse Direction +ve?"=TRUE, "Time offset"=0, "Amplitude offset"=0.0}, {"Start"=13792, "End"=13859, "Impulse Plane"=enum."Yaw", "Impulse Direction +ve?"=FALSE, "Time offset"=0, "Amplitude offset"=0.0}, {"Start"=21067, "End"=21133, "Impulse Plane"=enum."LARP", "Impulse Direction +ve?"=FALSE, "Time offset"=0, "Amplitude offset"=0.0}, {"Start"=21602, "End"=21667, "Impulse Plane"=enum."LARP", "Impulse Direction +ve?"=FALSE, "Time offset"=0, "Amplitude offset"=0.0}, {"Start"=22324, "End"=22386, "Impulse Plane"=enum."LARP", "Impulse Direction +ve?"=FALSE, "Time offset"=0, "Amplitude offset"=0.0}, {"Start"=23277, "End"=23335, "Impulse Plane"=enum."LARP", "Impulse Direction +ve?"=TRUE, "Time offset"=0, "Amplitude offset"=0.0}, {"Start"=24381, "End"=24445, "Impulse Plane"=enum."LARP", "Impulse Direction +ve?"=FALSE, "Time offset"=0, "Amplitude offset"=0.0}, {"Start"=24921, "End"=24983, "Impulse Plane"=enum."LARP", "Impulse Direction +ve?"=FALSE, "Time offset"=0, "Amplitude offset"=0.0}, {"Start"=27314, "End"=27375, "Impulse Plane"=enum."LARP", "Impulse Direction +ve?"=TRUE, "Time offset"=0, "Amplitude offset"=0.0}, {"Start"=29052, "End"=29115, "Impulse Plane"=enum."LARP", "Impulse Direction +ve?"=TRUE, "Time offset"=0, "Amplitude offset"=0.0}, {"Start"=30775, "End"=30838, "Impulse Plane"=enum."LARP", "Impulse Direction +ve?"=TRUE, "Time offset"=0, "Amplitude offset"=0.0}, {"Start"=31466, "End"=31529, "Impulse Plane"=enum."LARP", "Impulse Direction +ve?"=FALSE, "Time offset"=0, "Amplitude offset"=0.0}, {"Start"=31937, "End"=32000, "Impulse Plane"=enum."LARP", "Impulse Direction +ve?"=FALSE, "Time offset"=0, "Amplitude offset"=0.0}, {"Start"=33057, "End"=33118, "Impulse Plane"=enum."LARP", "Impulse Direction +ve?"=TRUE, "Time offset"=0, "Amplitude offset"=0.0}, {"Start"=33554, "End"=33613, "Impulse Plane"=enum."LARP", "Impulse Direction +ve?"=TRUE, "Time offset"=0, "Amplitude offset"=0.0}, {"Start"=35880, "End"=35943, "Impulse Plane"=enum."LARP", "Impulse Direction +ve?"=FALSE, "Time offset"=0, "Amplitude offset"=0.0}, {"Start"=36452, "End"=36513, "Impulse Plane"=enum."LARP", "Impulse Direction +ve?"=TRUE, "Time offset"=0, "Amplitude offset"=0.0}, {"Start"=36992, "End"=37057, "Impulse Plane"=enum."LARP", "Impulse Direction +ve?"=TRUE, "Time offset"=0, "Amplitude offset"=0.0}, {"Start"=38507, "End"=38572, "Impulse Plane"=enum."LARP", "Impulse Direction +ve?"=FALSE, "Time offset"=0, "Amplitude offset"=0.0}, {"Start"=38985, "End"=39048, "Impulse Plane"=enum."LARP", "Impulse Direction +ve?"=FALSE, "Time offset"=0, "Amplitude offset"=0.0}, {"Start"=48296, "End"=48359, "Impulse Plane"=enum."RALP", "Impulse Direction +ve?"=TRUE, "Time offset"=0, "Amplitude offset"=0.0}, {"Start"=48749, "End"=48812, "Impulse Plane"=enum."RALP", "Impulse Direction +ve?"=TRUE, "Time offset"=0, "Amplitude offset"=0.0}, {"Start"=49738, "End"=49797, "Impulse Plane"=enum."RALP", "Impulse Direction +ve?"=FALSE, "Time offset"=0, "Amplitude offset"=0.0}, {"Start"=52058, "End"=52118, "Impulse Plane"=enum."RALP", "Impulse Direction +ve?"=TRUE, "Time offset"=0, "Amplitude offset"=0.0}, {"Start"=52977, "End"=53037, "Impulse Plane"=enum."Roll", "Impulse Direction +ve?"=FALSE, "Time offset"=0, "Amplitude offset"=0.0}, {"Start"=55148, "End"=55210, "Impulse Plane"=enum."RALP", "Impulse Direction +ve?"=FALSE, "Time offset"=0, "Amplitude offset"=0.0}, {"Start"=55897, "End"=55958, "Impulse Plane"=enum."RALP", "Impulse Direction +ve?"=FALSE, "Time offset"=0, "Amplitude offset"=0.0}, {"Start"=57554, "End"=57621, "Impulse Plane"=enum."RALP", "Impulse Direction +ve?"=FALSE, "Time offset"=0, "Amplitude offset"=0.0}, {"Start"=58201, "End"=58264, "Impulse Plane"=enum."RALP", "Impulse Direction +ve?"=TRUE, "Time offset"=0, "Amplitude offset"=0.0}, {"Start"=58741, "End"=58807, "Impulse Plane"=enum."RALP", "Impulse Direction +ve?"=TRUE, "Time offset"=0, "Amplitude offset"=0.0}, {"Start"=59293, "End"=59356, "Impulse Plane"=enum."RALP", "Impulse Direction +ve?"=TRUE, "Time offset"=0, "Amplitude offset"=0.0}, {"Start"=60285, "End"=60344, "Impulse Plane"=enum."RALP", "Impulse Direction +ve?"=TRUE, "Time offset"=0, "Amplitude offset"=0.0}, {"Start"=60770, "End"=60836, "Impulse Plane"=enum."RALP", "Impulse Direction +ve?"=FALSE, "Time offset"=0, "Amplitude offset"=0.0}, {"Start"=61296, "End"=61356, "Impulse Plane"=enum."RALP", "Impulse Direction +ve?"=TRUE, "Time offset"=0, "Amplitude offset"=0.0}, {"Start"=62086, "End"=62148, "Impulse Plane"=enum."RALP", "Impulse Direction +ve?"=FALSE, "Time offset"=0, "Amplitude offset"=0.0}, {"Start"=64473, "End"=64534, "Impulse Plane"=enum."RALP", "Impulse Direction +ve?"=TRUE, "Time offset"=0, "Amplitude offset"=0.0}, {"Start"=65000, "End"=65065, "Impulse Plane"=enum."RALP", "Impulse Direction +ve?"=TRUE, "Time offset"=0, "Amplitude offset"=0.0}, {"Start"=81835, "End"=81899, "Impulse Plane"=enum."Pitch", "Impulse Direction +ve?"=TRUE, "Time offset"=0, "Amplitude offset"=0.0}, {"Start"=82298, "End"=82361, "Impulse Plane"=enum."Pitch", "Impulse Direction +ve?"=TRUE, "Time offset"=0, "Amplitude offset"=0.0}, {"Start"=82763, "End"=82825, "Impulse Plane"=enum."Pitch", "Impulse Direction +ve?"=TRUE, "Time offset"=0, "Amplitude offset"=0.0}, {"Start"=83203, "End"=83268, "Impulse Plane"=enum."Pitch", "Impulse Direction +ve?"=TRUE, "Time offset"=0, "Amplitude offset"=0.0}, {"Start"=85375, "End"=85436, "Impulse Plane"=enum."RALP", "Impulse Direction +ve?"=FALSE, "Time offset"=0, "Amplitude offset"=0.0}, {"Start"=87235, "End"=87300, "Impulse Plane"=enum."Pitch", "Impulse Direction +ve?"=TRUE, "Time offset"=0, "Amplitude offset"=0.0}, {"Start"=87823, "End"=87888, "Impulse Plane"=enum."Pitch", "Impulse Direction +ve?"=TRUE, "Time offset"=0, "Amplitude offset"=0.0}, {"Start"=88302, "End"=88363, "Impulse Plane"=enum."Pitch", "Impulse Direction +ve?"=TRUE, "Time offset"=0, "Amplitude offset"=0.0}, {"Start"=88696, "End"=88759, "Impulse Plane"=enum."Pitch", "Impulse Direction +ve?"=TRUE, "Time offset"=0, "Amplitude offset"=0.0}, {"Start"=89143, "End"=89209, "Impulse Plane"=enum."Pitch", "Impulse Direction +ve?"=TRUE, "Time offset"=0, "Amplitude offset"=0.0}, {"Start"=92014, "End"=92080, "Impulse Plane"=enum."Pitch", "Impulse Direction +ve?"=FALSE, "Time offset"=0, "Amplitude offset"=0.0}, {"Start"=93822, "End"=93885, "Impulse Plane"=enum."Pitch", "Impulse Direction +ve?"=TRUE, "Time offset"=0, "Amplitude offset"=0.0}, {"Start"=94647, "End"=94711, "Impulse Plane"=enum."Pitch", "Impulse Direction +ve?"=TRUE, "Time offset"=0, "Amplitude offset"=0.0}, {"Start"=95049, "End"=95112, "Impulse Plane"=enum."Pitch", "Impulse Direction +ve?"=TRUE, "Time offset"=0, "Amplitude offset"=0.0}, {"Start"=95915, "End"=95977, "Impulse Plane"=enum."RALP", "Impulse Direction +ve?"=TRUE, "Time offset"=0, "Amplitude offset"=0.0}, {"Start"=96746, "End"=96813, "Impulse Plane"=enum."Pitch", "Impulse Direction +ve?"=FALSE, "Time offset"=0, "Amplitude offset"=0.0}, {"Start"=100931, "End"=100992, "Impulse Plane"=enum."Roll", "Impulse Direction +ve?"=FALSE, "Time offset"=0, "Amplitude offset"=0.0}, {"Start"=101345, "End"=101407, "Impulse Plane"=enum."Roll", "Impulse Direction +ve?"=FALSE, "Time offset"=0, "Amplitude offset"=0.0}, {"Start"=101816, "End"=101877, "Impulse Plane"=enum."Roll", "Impulse Direction +ve?"=FALSE, "Time offset"=0, "Amplitude offset"=0.0}, {"Start"=102703, "End"=102766, "Impulse Plane"=enum."Roll", "Impulse Direction +ve?"=FALSE, "Time offset"=0, "Amplitude offset"=0.0}, {"Start"=103702, "End"=103768, "Impulse Plane"=enum."Roll", "Impulse Direction +ve?"=TRUE, "Time offset"=0, "Amplitude offset"=0.0}, {"Start"=104182, "End"=104243, "Impulse Plane"=enum."Roll", "Impulse Direction +ve?"=FALSE, "Time offset"=0, "Amplitude offset"=0.0}, {"Start"=105630, "End"=105691, "Impulse Plane"=enum."Roll", "Impulse Direction +ve?"=FALSE, "Time offset"=0, "Amplitude offset"=0.0}, {"Start"=106122, "End"=106186, "Impulse Plane"=enum."Roll", "Impulse Direction +ve?"=TRUE, "Time offset"=0, "Amplitude offset"=0.0}, {"Start"=106547, "End"=106606, "Impulse Plane"=enum."Roll", "Impulse Direction +ve?"=FALSE, "Time offset"=0, "Amplitude offset"=0.0}, {"Start"=106964, "End"=107027, "Impulse Plane"=enum."Roll", "Impulse Direction +ve?"=FALSE, "Time offset"=0, "Amplitude offset"=0.0}, {"Start"=107830, "End"=107892, "Impulse Plane"=enum."Roll", "Impulse Direction +ve?"=FALSE, "Time offset"=0, "Amplitude offset"=0.0}, {"Start"=108543, "End"=108605, "Impulse Plane"=enum."Roll", "Impulse Direction +ve?"=FALSE, "Time offset"=0, "Amplitude offset"=0.0}, {"Start"=108953, "End"=109019, "Impulse Plane"=enum."Roll", "Impulse Direction +ve?"=FALSE, "Time offset"=0, "Amplitude offset"=0.0}, {"Start"=110057, "End"=110126, "Impulse Plane"=enum."Roll", "Impulse Direction +ve?"=TRUE, "Time offset"=0, "Amplitude offset"=0.0}, {"Start"=110555, "End"=110617, "Impulse Plane"=enum."Roll", "Impulse Direction +ve?"=FALSE, "Time offset"=0, "Amplitude offset"=0.0}, {"Start"=111408, "End"=111474, "Impulse Plane"=enum."Roll", "Impulse Direction +ve?"=FALSE, "Time offset"=0, "Amplitude offset"=0.0}, {"Start"=112383, "End"=112447, "Impulse Plane"=enum."Roll", "Impulse Direction +ve?"=FALSE, "Time offset"=0, "Amplitude offset"=0.0}, {"Start"=112817, "End"=112884, "Impulse Plane"=enum."Roll", "Impulse Direction +ve?"=FALSE, "Time offset"=0, "Amplitude offset"=0.0}, {"Start"=113289, "End"=113355, "Impulse Plane"=enum."Roll", "Impulse Direction +ve?"=TRUE, "Time offset"=0, "Amplitude offset"=0.0}, {"Start"=113771, "End"=113838, "Impulse Plane"=enum."Roll", "Impulse Direction +ve?"=FALSE, "Time offset"=0, "Amplitude offset"=0.0}, {"Start"=114303, "End"=114368, "Impulse Plane"=enum."Roll", "Impulse Direction +ve?"=FALSE, "Time offset"=0, "Amplitude offset"=0.0}, {"Start"=114726, "End"=114791, "Impulse Plane"=enum."Roll", "Impulse Direction +ve?"=FALSE, "Time offset"=0, "Amplitude offset"=0.0}, {"Start"=115183, "End"=115247, "Impulse Plane"=enum."Roll", "Impulse Direction +ve?"=FALSE, "Time offset"=0, "Amplitude offset"=0.0}] {"Amplitude offset" format="%.2f"}, 9 "Impulse Data":T3={"Data Channels"=[], "Sample Rate"=250, "Channel List"=["Hx Position-in-Head", "Hy Position-in-Head", "Hz Position-in-Head", "Hx Velocity-in-Head", "Hy Velocity-in-Head", "Hz Velocity-in-Head", "Hl Velocity-in-Head", "Hr Velocity-in-Head", "Lx Position-in-Head", "Ly Position-in-Head", "Lz Position-in-Head", "Lx Velocity-in-Head", "Ly Velocity-in-Head", "Lz Velocity-in-Head", "Ll Velocity-in-Head", "Lr Velocity-in-Head", "Rx Position-in-Head", "Ry Position-in-Head", "Rz Position-in-Head", "Rx Velocity-in-Head", "Ry Velocity-in-Head", "Rz Velocity-in-Head", "Rl Velocity-in-Head", "Rr Velocity-in-Head", "Button", "Ascension X", "Ascension X Vel", "Ascension Y", "Ascension Y Vel", "Ascension Z", "Ascension Z Vel", " "]} {"Data Channels" format="%.2f"}) -> ()   [LabVIEW 2016, in "generate report.lvlib"]
uses:
  generate report.lvlib
  comm/impulse/impulse functions.lvlib
panel:
  in  "Means":bool
  in  "Target Position":T1(ring)
  in  "Subject ID":enum16{"dsz", "nbs", "jpc", "aam", "mcs", "rac"}(ring)
  in  "Save to File":bool
  in  "stop":bool
  # "Copyright Americo A. Migliaccio (c) 2002 All Rights Reserved by Author"
  # "-"
  # "+"
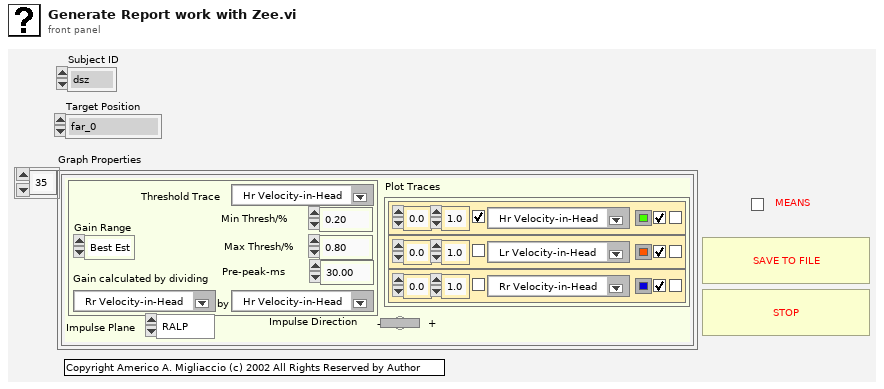
[diagram p1: front panel]
types:
  T1 = enum16{"far_0", "far_left_20", "far_left_30", "far_right_20", "far_right_30", "near_0", "near_left_20", "near_right_20"}
  T2 = cluster{"Plot Traces":cluster{"Color Box":u32, "Boolean":bool, "List 2":u16, "Boolean 2":bool, "Boolean 3":bool, "Offset":dbl, "Gain":dbl}[], "Gain Calculations":cluster{"Threshold Trace":u16, "Min Thresh/%":dbl, "Max Thresh/%":dbl, "Gain calculated by dividing":u16, "Gain Range":enum16{"Peak %", "Best Est", "Thresh"}, "Pre-peak-ms":dbl, "by":u16}, "Impulse Plane":enum16{"Other", "Yaw", "Pitch", "Roll", "LARP", "RALP"}, "Impulse Direction":bool}[]
  T3 = cluster{"Data Channels":dbl[][], "Sample Rate":i32, "Channel List":string[]}
  T4 = cluster{"Start":i32, "End":i32, "Impulse Plane":enum16{"Other", "Yaw", "Pitch", "Roll", "LARP", "RALP"}, "Impulse Direction +ve?":bool, "Time offset":i32, "Amplitude offset":dbl}[]
  T5 = enum16{"open", "open or create", "create or replace", "create", "open (read only)"}
  T6 = enum16{"Other", "Yaw", "Pitch", "Roll", "LARP", "RALP"}
  T7 = cluster{"Color Box":u32, "Boolean":bool, "List 2":u16, "Boolean 2":bool, "Boolean 3":bool, "Offset":dbl, "Gain":dbl}[]
  T8 = cluster{"Threshold Trace":u16, "Min Thresh/%":dbl, "Max Thresh/%":dbl, "Gain calculated by dividing":u16, "Gain Range":enum16{"Peak %", "Best Est", "Thresh"}, "Pre-peak-ms":dbl, "by":u16}
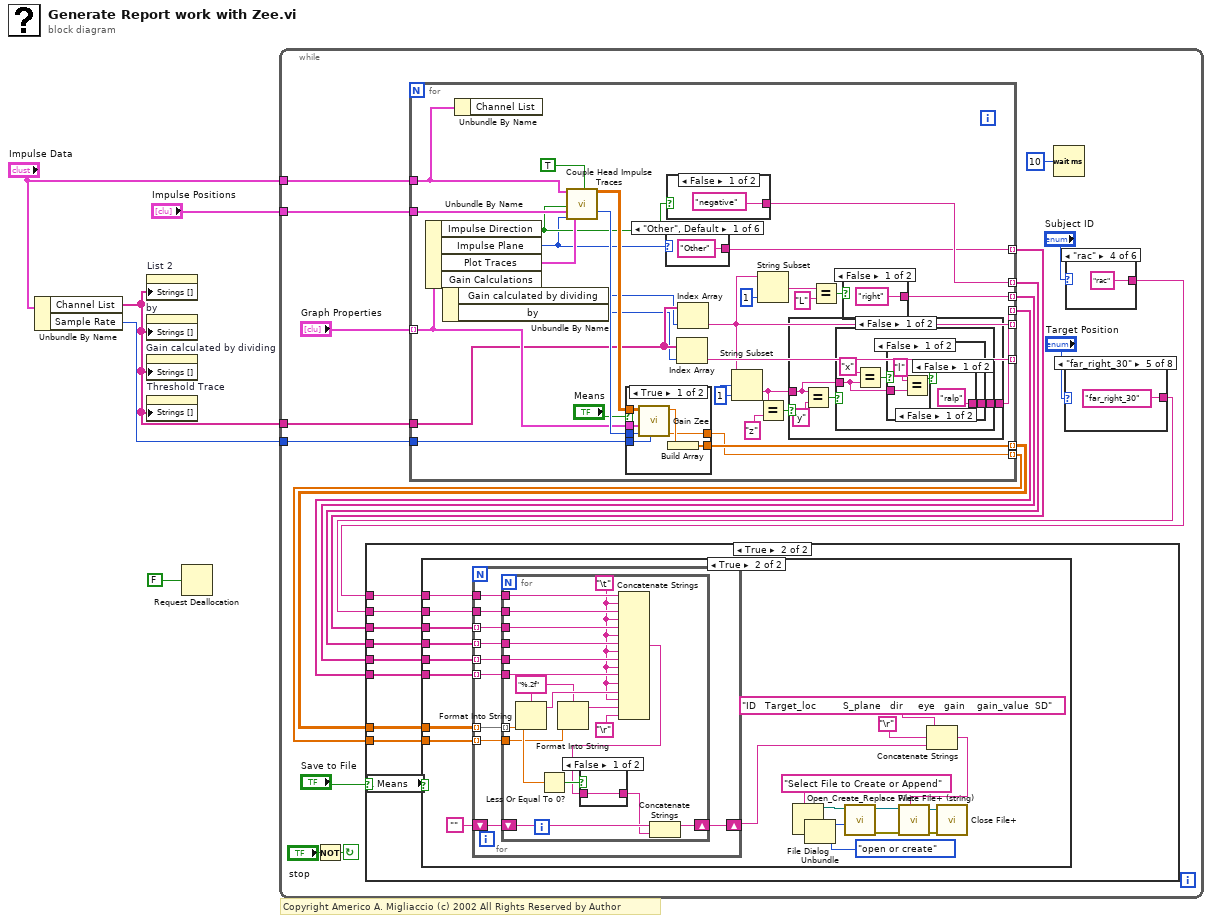
[diagram p0: block diagram]
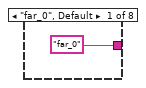
[diagram p2: hidden frame]
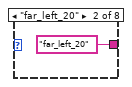
[diagram p3: hidden frame]
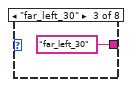
[diagram p4: hidden frame]
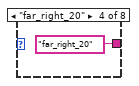
[diagram p5: hidden frame]
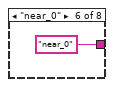
[diagram p6: hidden frame]
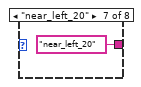
[diagram p7: hidden frame]
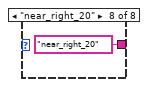
[diagram p8: hidden frame]
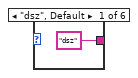
[diagram p9: hidden frame]
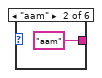
[diagram p10: hidden frame]
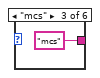
[diagram p11: hidden frame]
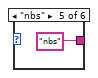
[diagram p12: hidden frame]
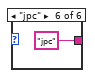
[diagram p13: hidden frame]
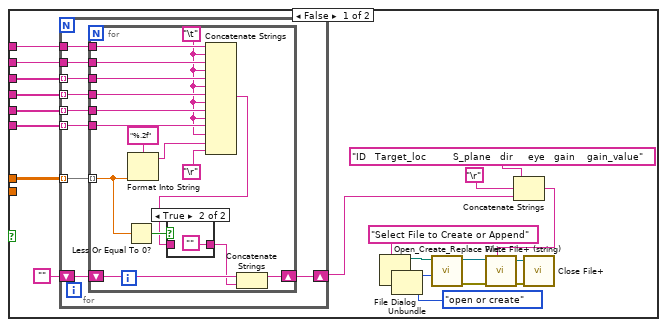
[diagram p15: hidden frame]
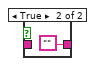
[diagram p17: hidden frame]
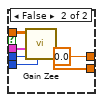
[diagram p18: hidden frame]
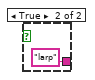
[diagram p19: hidden frame]
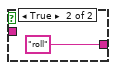
[diagram p20: hidden frame]
diagram:
  # "Copyright Americo A. Migliaccio (c) 2002 All Rights Reserved by Author"
  n1 = Unbundle By Name("Impulse Data") -> ("Channel List"=w2:string[], "Sample Rate"=w4:i32)
  n2 = property on="List 2" class="Ring (strict)"("Strings []"=w2) -> ()  [unwired: 2 in, 2 out]
  n3 = property on="by" class="Ring (strict)"("Strings []"=w2) -> ()  [unwired: 2 in, 2 out]
  n4 = property on="Gain calculated by dividing" class="Ring (strict)"("Strings []"=w2) -> ()  [unwired: 2 in, 2 out]
  n5 = property on="Threshold Trace" class="Ring (strict)"("Strings []"=w2) -> ()  [unwired: 2 in, 2 out]
  n6 = Request Deallocation(FALSE ("flag")) -> ()
  n7 = while {
    tunnel: w4 -> [w22]
    tunnel: "Impulse Positions" -> [w23]
    tunnel: "Impulse Data" -> [w24]
    tunnel: w2 -> [w18]
    stop <- w19 continue-if-true
    n8 = Not(x="stop") -> (.not. x?=w19:bool)
    n9 = for {
      tunnel: "Graph Properties" -> [w172] mode=indexing
      tunnel: w23 -> [w176]
      tunnel: w24 -> [w169]
      tunnel: w22 -> [w171]
      tunnel: [w159] -> w17 mode=indexing
      tunnel: w18 -> [w167]
      tunnel: [w154] -> _ mode=indexing
      tunnel: [w164] -> _ mode=indexing
      tunnel: [w162] -> w14 mode=indexing
      tunnel: [w161] -> w13 mode=indexing
      tunnel: [w155] -> w8 mode=indexing
      tunnel: [w148] -> w7 mode=indexing
      tunnel: [w147] -> w6 mode=indexing
      w153 = 1 ("length (rest)")
      n10 = Unbundle By Name(w172) -> ("Impulse Direction"=w163:bool, "Impulse Plane"=w160:T6, "Plot Traces"=w173:T7, "Gain Calculations"=w168:T8)
      n11 = Unbundle By Name(w168) -> ("Gain calculated by dividing"=w166:u16, "by"=w165:u16)
      n12 = Unbundle By Name(w169) -> ()  [unwired: 1 out]
      n13 = call "Couple Head Impulse Traces.vi"("Data Input"=w169, "Impulse Positions"=w176, "Impulse Direction +ve?"=w163, "Impulse Plane"=w160, "Plot Selection 2"=w173, "Interpolate"=TRUE) -> ("No Impulses"=w174:i32, "Impulses"=w175:dbl[][])  [unwired: 10 in, 2 out]
      n14 = case shown="True" "Means" {
        tunnel: w175 -> [w183 w189]
        tunnel: w174 -> [w182 w188]
        tunnel: w172 -> [w181 w187]
        tunnel: w171 -> [w180 w186]
        tunnel: [w178 w185] -> w161
        tunnel: [w177 0.0 ("STD")] -> w147
        frame True {
          n15 = call "Gain Zee.vi"("Sample Rate"=w180, "Number of Impulses"=w182, "Graph Cluster"=w181, "Data (in)"=w183) -> ("STD"=w177:dbl, "GAIN"=w179:dbl)  [unwired: 3 in, 1 out]
          n16 = Build Array(w179) -> (w178:dbl[])
        }
        frame False {
          n17 = call "Gain Zee.vi"("Sample Rate"=w186, "Number of Impulses"=w188, "Graph Cluster"=w187, "Data (in)"=w189) -> ("STD array"=w185:dbl[])  [unwired: 3 in, 2 out]
        }
      }
      n18 = case shown="\"Other\", Default" w160 {
        tunnel: ["Other" "yaw" "pitch" "roll" "larp" "ralp"] -> w159
        frame "Other", Default {
        }
        frame "Yaw" {
        }
        frame "Pitch" {
        }
        frame "Roll" {
        }
        frame "LARP" {
        }
        frame "RALP" {
        }
      }
      n19 = case shown="False" w163 {
        tunnel: ["negative" "positive"] -> w162
        frame False {
        }
        frame True {
        }
      }
      n20 = Index Array(array=w167, index=w165) -> (element=w164:string)
      n21 = Index Array(array=w167, index=w166) -> (element=w154:string)
      n22 = String Subset(string=w154, offset (0)=w153, length (rest)=w153) -> (substring=w149:string)
      n23 = String Subset(string=w154, length (rest)=1 ("length (rest)")) -> (substring=w157:string)  [unwired: 1 in]
      n24 = Equal?(x=w149, y="z") -> (x = y?=w151:bool)
      n25 = case shown="False" w151 {
        tunnel: [w191 "hor"] -> w148
        tunnel: w149 -> [w190 _]
        frame False {
          n26 = Equal?(x=w190, y="y") -> (x = y?=w192:bool)
          n27 = case shown="False" w192 {
            tunnel: [w195 "pitch"] -> w191
            tunnel: w190 -> [w194 _]
            frame False {
              n28 = Equal?(x="x" ("y"), y=w194) -> (x = y?=w196:bool)
              n29 = case shown="False" w196 {
                tunnel: [w199 "roll"] -> w195
                tunnel: w194 -> [w201 _]
                frame False {
                  n30 = Equal?(x="l" ("y"), y=w201) -> (x = y?=w198:bool)
                  n31 = case shown="False" w198 {
                    tunnel: ["ralp" ("y") "larp" ("y")] -> w199
                    frame False {
                    }
                    frame True {
                    }
                  }
                }
                frame True {
                }
              }
            }
            frame True {
            }
          }
        }
        frame True {
        }
      }
      n32 = Equal?(x=w157, y="L") -> (x = y?=w152:bool)
      n33 = case shown="False" w152 {
        tunnel: ["right" "left"] -> w155
        frame False {
        }
        frame True {
        }
      }
    }
    n34 = Wait (ms)(milliseconds to wait=u32 10) -> ()  [unwired: 1 out]
    n35 = case shown="\"far_right_30\"" "Target Position" {
      tunnel: ["far_0" "far_left_20" "far_left_30" "far_right_20" "far_right_30" "near_0" "near_left_20" "near_right_20"] -> w10
      frame "far_0", Default {
      }
      frame "far_left_20" {
      }
      frame "far_left_30" {
      }
      frame "far_right_20" {
      }
      frame "far_right_30" {
      }
      frame "near_0" {
      }
      frame "near_left_20" {
      }
      frame "near_right_20" {
      }
    }
    n36 = case shown="\"rac\"" "Subject ID" {
      tunnel: ["dsz" "aam" "mcs" "rac" "nbs" "jpc"] -> w9
      frame "dsz", Default {
      }
      frame "aam" {
      }
      frame "mcs" {
      }
      frame "rac" {
      }
      frame "nbs" {
      }
      frame "jpc" {
      }
    }
    n37 = case shown="True" "Save to File" {
      tunnel: w17 -> [_ w47]
      tunnel: w14 -> [_ w46]
      tunnel: w13 -> [_ w45]
      tunnel: w10 -> [_ w43]
      tunnel: w9 -> [_ w44]
      tunnel: w8 -> [_ w42]
      tunnel: w7 -> [_ w41]
      tunnel: w6 -> [_ w40]
      frame False {
      }
      frame True {
        n38 = local read "Means"() -> (w39:bool)
        n39 = case shown="True" w39 {
          tunnel: w47 -> [w67 w115]
          tunnel: w46 -> [w54 w102]
          tunnel: w45 -> [w53 w101]
          tunnel: w44 -> [w52 w100]
          tunnel: w43 -> [w51 w99]
          tunnel: w42 -> [w50 w98]
          tunnel: w41 -> [w49 w97]
          tunnel: w40 -> [_ w96]
          frame False {
            n40 = for {
              tunnel: w67 -> [w76] mode=indexing
              shift-right: [w73] -> w55
              shift-left: "" -> [w74]
              tunnel: w54 -> [w75] mode=indexing
              tunnel: w53 -> [w72] mode=indexing
              tunnel: w52 -> [w71]
              tunnel: w51 -> [w70]
              tunnel: w50 -> [w69] mode=indexing
              tunnel: w49 -> [w68] mode=indexing
              n41 = for {
                tunnel: w76 -> [w83]
                tunnel: w75 -> [w84]
                shift-right: [w91] -> w73
                shift-left: w74 -> [w88]
                tunnel: w72 -> [w90] mode=indexing
                tunnel: w71 -> [w86]
                tunnel: w70 -> [w85]
                tunnel: w69 -> [w82]
                tunnel: w68 -> [w81]
                w80 = "\t"
                n42 = Less Or Equal To 0?(x=w90) -> (x <= 0?=w89:bool)
                n43 = Format Into String(format string="%.2f", w90) -> (resulting string=w77:string)  [unwired: 2 in, 1 out]
                n44 = Concatenate Strings(w86, w80, w85, w80, w83, w80, w84, w80, w82, w80, w81, w80, w77, "\r") -> (w79:string)
                n45 = case shown="True" w89 {
                  tunnel: w79 -> [w93 _]
                  tunnel: [w93 ""] -> w87
                  frame False {
                  }
                  frame True {
                  }
                }
                n46 = Concatenate Strings(w88, w87) -> (w91:string)
              }
            }
            n47 = File Dialog(7:"Select File to Create or Append" ("prompt")) -> (0:w48:errorcluster, 3:w63:path)  [unwired: 6 in, 2 out]
            n48 = Unbundle(w48) -> ()  [unwired: 3 out]
            n49 = call <vilib>:"Open_Create_Replace File.vi"("function (open:0)"=T5."open or create", "file path"=w63) -> ("error out"=w65:errorcluster, "refnum"=w64:refnum<file>)  [unwired: 6 in, 2 out]
            n50 = Concatenate Strings("ID   Target_loc         S_plane   dir     eye   gain    gain_value" ("prompt"), "\r", w55) -> (w59:string)
            n51 = call <vilib>:"Write File+ (string).vi"("string"=w59, "error in (no error)"=w65, "refnum"=w64) -> ("error out"=w61:errorcluster, "dup refnum"=w62:refnum<file>)  [unwired: 4 in, 1 out]
            n52 = call <vilib>:"Close File+.vi"("error in (no error)"=w61, "refnum"=w62) -> ()  [unwired: 3 in, 3 out]
          }
          frame True {
            n53 = for {
              tunnel: w115 -> [w125] mode=indexing
              shift-right: [w122] -> w103
              shift-left: "" -> [w123]
              tunnel: w102 -> [w124] mode=indexing
              tunnel: w101 -> [w121] mode=indexing
              tunnel: w100 -> [w120]
              tunnel: w99 -> [w119]
              tunnel: w98 -> [w118] mode=indexing
              tunnel: w97 -> [w117] mode=indexing
              tunnel: w96 -> [w116] mode=indexing
              n54 = for {
                tunnel: w125 -> [w135]
                tunnel: w124 -> [w136]
                shift-right: [w143] -> w122
                shift-left: w123 -> [w140]
                tunnel: w121 -> [w142] mode=indexing
                tunnel: w120 -> [w138]
                tunnel: w119 -> [w137]
                tunnel: w118 -> [w134]
                tunnel: w117 -> [w133]
                tunnel: w116 -> [w126]
                w130 = "\t"
                w128 = "%.2f" ("format string")
                n55 = Format Into String(format string=w128, w142) -> (resulting string=w131:string)  [unwired: 2 in, 1 out]
                n56 = Less Or Equal To 0?(x=w142) -> (x <= 0?=w141:bool)
                n57 = Format Into String(format string=w128, w126) -> (resulting string=w127:string)  [unwired: 2 in, 1 out]
                n58 = Concatenate Strings(w138, w130, w137, w130, w135, w130, w136, w130, w134, w130, w133, w130, w131, w130, w127, "\r") -> (w132:string)
                n59 = case shown="False" w141 {
                  tunnel: w132 -> [w144 _]
                  tunnel: [w144 ""] -> w139
                  frame False {
                  }
                  frame True {
                  }
                }
                n60 = Concatenate Strings(w140, w139) -> (w143:string)
              }
            }
            n61 = File Dialog(7:"Select File to Create or Append" ("prompt")) -> (0:w95:errorcluster, 3:w111:path)  [unwired: 6 in, 2 out]
            n62 = Unbundle(w95) -> ()  [unwired: 3 out]
            n63 = call <vilib>:"Open_Create_Replace File.vi"("function (open:0)"=T5."open or create", "file path"=w111) -> ("error out"=w113:errorcluster, "refnum"=w112:refnum<file>)  [unwired: 6 in, 2 out]
            n64 = Concatenate Strings("ID   Target_loc         S_plane   dir     eye   gain    gain_value  SD" ("prompt"), "\r", w103) -> (w107:string)
            n65 = call <vilib>:"Write File+ (string).vi"("string"=w107, "error in (no error)"=w113, "refnum"=w112) -> ("error out"=w109:errorcluster, "dup refnum"=w110:refnum<file>)  [unwired: 4 in, 1 out]
            n66 = call <vilib>:"Close File+.vi"("error in (no error)"=w109, "refnum"=w110) -> ()  [unwired: 3 in, 3 out]
          }
        }
      }
    }
  }
